vi "未命名 1.vi"() -> ()   [LabVIEW 2010]
uses:
  <vilib>/Instr/_visa.llb/VISA Configure Serial Port (Instr).vi
panel:
  in  "写入缓冲区":string
  in  "Input\nbuffer size":u32=4096
  in  "flow control":u16(ring) items=["None"=0, "XON/XOFF"=1, "RTS/CTS"=2, "DTR/DSR"=4]
  in  "timeout (ms)":u32=10000
  in  "stop bits":u16(ring)=10 items=["1.0"=10, "1.5"=15, "2.0"=20]
  in  "parity":u16(ring) items=["None", "Odd", "Even", "Mark", "Space"]
  in  "data bits":u16=8 min=5 max=8 step=1
  in  "VISA resource name":refnum<visa-resource-name>="COM1"
  in  "baud rate":u32=9600
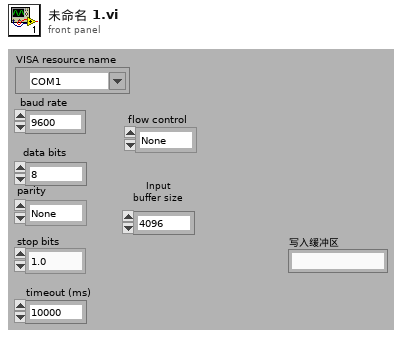
[diagram p1: front panel]
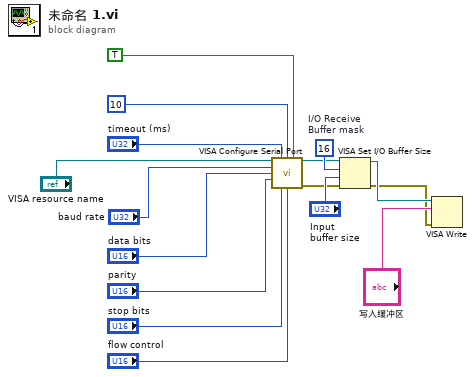
[diagram p0: block diagram]
diagram:
  w7 = u16 16  # I/O Receive Buffer mask
  n1 = call-poly "VISA Configure Serial Port"("VISA resource name"="VISA resource name", "timeout (10sec)"="timeout (ms)", "termination char\n(0xA = '\\n' = LF)"=u8 10 ("termination char\n(0xA = '\\n' = LF)"), "Enable Termination\nChar (T)"=TRUE ("End read on termination character?"), "baud rate (9600)"="baud rate", "data bits (8)"="data bits", "parity (0:none)"="parity", "stop bits (10: 1 bit)"="stop bits", "flow control (0:none)"="flow control") -> ("VISA resource name out"=w6:refnum<visa-resource-name>, "error out"=w4:errorcluster)  [unwired: 1 in, 4 out]
  n2 = VISA Set I/O Buffer Size(VISA resource name=w6, mask (16)=w7, size (4096)="Input\nbuffer size", error in (no error)=w4) -> (VISA resource name out=w2:refnum<visa-resource-name>, error out=w1:errorcluster)
  n3 = VISA Write(VISA resource name=w2, write buffer="写入缓冲区", error in (no error)=w1) -> ()  [unwired: 3 out]
